vi "Debugger_Application.vi"() -> ()   [LabVIEW 2016]
uses:
  Z:/original_project/CodeConverter/Controls/CommandLine.ctl
  Z:/original_project/CodeConverter/Controls/EX.Command.ctl
  Z:/original_project/CodeConverter/Controls/WB.Operation.ctl
  Z:/original_project/CodeConverter/SoftCoreCodeConverter.lvlib
panel:
  out "Instruction stop":bool
  in  "Breakpoint signal":bool
  in  "Breakpoint control":i32
  in  "Run":bool
  out "Instruction Number":i32=7
  in  "Breakpoint On/Off":bool
  in  "Instruction Step Mode":bool
  in  "Instruction  Delay":u32=100
  out "Current Output /Ins":dbl
  out "DataMemory Out":dbl[](array[numeric])=[0.0, 1.0, 2.0, 3.0, 4.0, 5.0, 6.0, 7.0, 8.0, 9.0, 10.0, 11.0, 15.0, 16.0, 17.0, 18.0, 19.0, 20.0, 0.0, 0.0, 0.0, 0.0, 0.0, 0.0, 0.0, 0.0, 0.0, 0.0, 0.0, 0.0, 0.0, 0.0, 0.0, 0.0, 0.0, 0.0, 0.0, 0.0, 0.0, 0.0, 0.0, 0.0, 0.0, 0.0, 0.0, 0.0, 0.0, 0.0, 0.0, 0.0, 0.0, 0.0, 0.0, 0.0, 0.0, 0.0, 0.0, 0.0, 0.0, 0.0, 0.0, 0.0, 0.0, 0.0, 0.0, 0.0, 0.0, 0.0, 0.0, 0.0, 0.0, 0.0, 0.0, 0.0, 0.0, 0.0, 0.0, 0.0, 0.0, 0.0, 0.0, 0.0, 0.0, 0.0, 0.0, 0.0, 0.0, 0.0, 0.0, 0.0, 0.0, 0.0, 0.0, 0.0, 0.0, 0.0, 0.0, 0.0, 0.0, 0.0, 0.0, 0.0, 0.0, 0.0, 0.0, 0.0, 0.0, 0.0, 0.0, 0.0, 0.0, 0.0, 0.0, 0.0, 0.0, 0.0, 0.0, 0.0, 0.0, 0.0, 0.0, 0.0, 0.0, 0.0, 0.0, 0.0, 0.0, 0.0, 0.0, 0.0, 0.0, 0.0, 0.0, 0.0, 0.0, 0.0, 0.0, 0.0, 0.0, 0.0, 0.0, 0.0, 0.0, 0.0, 0.0, 0.0, 0.0, 0.0, 0.0, 0.0, 0.0, 0.0, 0.0, 0.0, 0.0, 0.0, 0.0, 0.0, 0.0, 0.0, 0.0, 0.0, 0.0, 0.0, 0.0, 0.0, 0.0, 0.0, 0.0, 0.0, 0.0, 0.0, 0.0, 0.0, 0.0, 0.0, 0.0, 0.0, 0.0, 0.0, 0.0, 0.0, 0.0, 0.0, 0.0, 0.0, 0.0, 0.0, 0.0, 0.0, 0.0, 0.0, 0.0, 0.0, 0.0, 0.0, 0.0, 0.0, 0.0, 0.0, 0.0, 0.0, 0.0, 0.0, 0.0, 0.0, 0.0, 0.0, 0.0, 0.0, 0.0, 0.0, 0.0, 0.0, 0.0, 0.0, 0.0, 0.0, 0.0, 0.0, 0.0, 0.0, 0.0, 0.0, 0.0, 0.0, 0.0, 0.0, 0.0, 0.0, 0.0, 0.0, 0.0, 0.0, 0.0, 0.0, 0.0, 0.0, 0.0, 0.0, 0.0, 0.0, 0.0, 0.0, 0.0, 0.0, 0.0, 0.0, 0.0, 0.0, 0.0, 0.0, 0.0, 0.0, 0.0]
  out "Current Operation":T1=enum."None"
  out "Output array":dbl[](array[numeric])
  in  "Input":dbl[](array[numeric])=[0.0, 15.0, 20.0, 3.0, 4.0, 5.0, 6.0, 7.0, 8.0, 9.0, 10.0, 11.0, 15.0, 16.0, 17.0, 18.0, 19.0, 20.0, 0.0, 0.0, 0.0, 0.0, 0.0, 0.0, 0.0, 0.0, 0.0, 0.0, 0.0, 0.0, 0.0, 0.0, 0.0, 0.0, 0.0, 0.0, 0.0, 0.0, 0.0, 0.0, 0.0, 0.0, 0.0, 0.0, 0.0, 0.0, 0.0, 0.0, 0.0, 0.0, 0.0, 0.0, 0.0, 0.0, 0.0, 0.0, 0.0, 0.0, 0.0, 0.0, 0.0, 0.0, 0.0, 0.0, 0.0, 0.0, 0.0, 0.0, 0.0, 0.0, 0.0, 0.0, 0.0, 0.0, 0.0, 0.0, 0.0, 0.0, 0.0, 0.0, 0.0, 0.0, 0.0, 0.0, 0.0, 0.0, 0.0, 0.0, 0.0, 0.0, 0.0, 0.0, 0.0, 0.0, 0.0, 0.0, 0.0, 0.0, 0.0, 0.0, 0.0, 0.0, 0.0, 0.0, 0.0, 0.0, 0.0, 0.0, 0.0, 0.0, 0.0, 0.0, 0.0, 0.0, 0.0, 0.0, 0.0, 0.0, 0.0, 0.0, 0.0, 0.0, 0.0, 0.0, 0.0, 0.0, 0.0, 0.0, 0.0, 0.0, 0.0, 0.0, 0.0, 0.0, 0.0, 0.0, 0.0, 0.0, 0.0, 0.0, 0.0, 0.0, 0.0, 0.0, 0.0, 0.0, 0.0, 0.0, 0.0, 0.0, 0.0, 0.0, 0.0, 0.0, 0.0, 0.0, 0.0, 0.0, 0.0, 0.0, 0.0, 0.0, 0.0, 0.0, 0.0, 0.0, 0.0, 0.0, 0.0, 0.0, 0.0, 0.0, 0.0, 0.0, 0.0, 0.0, 0.0, 0.0, 0.0, 0.0, 0.0, 0.0, 0.0, 0.0, 0.0, 0.0, 0.0, 0.0, 0.0, 0.0, 0.0, 0.0, 0.0, 0.0, 0.0, 0.0, 0.0, 0.0, 0.0, 0.0, 0.0, 0.0, 0.0, 0.0, 0.0, 0.0, 0.0, 0.0, 0.0, 0.0, 0.0, 0.0, 0.0, 0.0, 0.0, 0.0, 0.0, 0.0, 0.0, 0.0, 0.0, 0.0, 0.0, 0.0, 0.0, 0.0, 0.0, 0.0, 0.0, 0.0, 0.0, 0.0, 0.0, 0.0, 0.0, 0.0, 0.0, 0.0, 0.0, 0.0, 0.0, 0.0, 0.0, 0.0, 0.0, 0.0, 0.0, 0.0, 0.0, 0.0, 0.0, 0.0, 0.0, 0.0, 0.0]
  out "Loop Mode Iteration":i32
  in  "Loop Delay":u32=1000
  in  "Loop Step Mode":bool
  in  "Loop Mode":bool
  in  "DataMemory Input":dbl[](array[numeric])=[0.0, 1.0, 2.0, 3.0, 4.0, 5.0, 6.0, 7.0, 8.0, 9.0, 10.0, 11.0, 15.0, 16.0, 17.0, 18.0, 19.0, 20.0, 0.0, 0.0, 0.0, 0.0, 0.0, 0.0, 0.0, 0.0, 0.0, 0.0, 0.0, 0.0, 0.0, 0.0, 0.0, 0.0, 0.0, 0.0, 0.0, 0.0, 0.0, 0.0, 0.0, 0.0, 0.0, 0.0, 0.0, 0.0, 0.0, 0.0, 0.0, 0.0, 0.0, 0.0, 0.0, 0.0, 0.0, 0.0, 0.0, 0.0, 0.0, 0.0, 0.0, 0.0, 0.0, 0.0, 0.0, 0.0, 0.0, 0.0, 0.0, 0.0, 0.0, 0.0, 0.0, 0.0, 0.0, 0.0, 0.0, 0.0, 0.0, 0.0, 0.0, 0.0, 0.0, 0.0, 0.0, 0.0, 0.0, 0.0, 0.0, 0.0, 0.0, 0.0, 0.0, 0.0, 0.0, 0.0, 0.0, 0.0, 0.0, 0.0, 0.0, 0.0, 0.0, 0.0, 0.0, 0.0, 0.0, 0.0, 0.0, 0.0, 0.0, 0.0, 0.0, 0.0, 0.0, 0.0, 0.0, 0.0, 0.0, 0.0, 0.0, 0.0, 0.0, 0.0, 0.0, 0.0, 0.0, 0.0, 0.0, 0.0, 0.0, 0.0, 0.0, 0.0, 0.0, 0.0, 0.0, 0.0, 0.0, 0.0, 0.0, 0.0, 0.0, 0.0, 0.0, 0.0, 0.0, 0.0, 0.0, 0.0, 0.0, 0.0, 0.0, 0.0, 0.0, 0.0, 0.0, 0.0, 0.0, 0.0, 0.0, 0.0, 0.0, 0.0, 0.0, 0.0, 0.0, 0.0, 0.0, 0.0, 0.0, 0.0, 0.0, 0.0, 0.0, 0.0, 0.0, 0.0, 0.0, 0.0, 0.0, 0.0, 0.0, 0.0, 0.0, 0.0, 0.0, 0.0, 0.0, 0.0, 0.0, 0.0, 0.0, 0.0, 0.0, 0.0, 0.0, 0.0, 0.0, 0.0, 0.0, 0.0, 0.0, 0.0, 0.0, 0.0, 0.0, 0.0, 0.0, 0.0, 0.0, 0.0, 0.0, 0.0, 0.0, 0.0, 0.0, 0.0, 0.0, 0.0, 0.0, 0.0, 0.0, 0.0, 0.0, 0.0, 0.0, 0.0, 0.0, 0.0, 0.0, 0.0, 0.0, 0.0, 0.0, 0.0, 0.0, 0.0, 0.0, 0.0, 0.0, 0.0, 0.0, 0.0, 0.0, 0.0, 0.0, 0.0, 0.0, 0.0, 0.0, 0.0, 0.0, 0.0, 0.0]
  in  "CoreCode":T2[][](array[typedef])=[[{"Ex.Command"=enum."None", "Ex.AddressIn1"=1.0, "Ex.AddressIn2"=0.0, "WB.Command"=enum."In", "WB.AddressOut"=3.0, "Bypass1"=0.0, "Bypass 2"=0.0}], [{"Ex.Command"=enum."None", "Ex.AddressIn1"=2.0, "Ex.AddressIn2"=0.0, "WB.Command"=enum."In", "WB.AddressOut"=4.0, "Bypass1"=0.0, "Bypass 2"=0.0}], [{"Ex.Command"=enum."None", "Ex.AddressIn1"=3.0, "Ex.AddressIn2"=4.0, "WB.Command"=enum."Mul", "WB.AddressOut"=5.0, "Bypass1"=0.0, "Bypass 2"=0.0}], [{"Ex.Command"=enum."None", "Ex.AddressIn1"=5.0, "Ex.AddressIn2"=0.0, "WB.Command"=enum."Mov", "WB.AddressOut"=6.0, "Bypass1"=0.0, "Bypass 2"=0.0}], [{"Ex.Command"=enum."None", "Ex.AddressIn1"=6.0, "Ex.AddressIn2"=0.0, "WB.Command"=enum."Out", "WB.AddressOut"=3.0, "Bypass1"=0.0, "Bypass 2"=0.0}], [{"Ex.Command"=enum."None", "Ex.AddressIn1"=0.0, "Ex.AddressIn2"=0.0, "WB.Command"=enum."None", "WB.AddressOut"=0.0, "Bypass1"=0.0, "Bypass 2"=0.0}], [{"Ex.Command"=enum."None", "Ex.AddressIn1"=0.0, "Ex.AddressIn2"=0.0, "WB.Command"=enum."None", "WB.AddressOut"=0.0, "Bypass1"=0.0, "Bypass 2"=0.0}], [{"Ex.Command"=enum."None", "Ex.AddressIn1"=5.0, "Ex.AddressIn2"=9.0, "WB.Command"=enum."None", "WB.AddressOut"=0.0, "Bypass1"=0.0, "Bypass 2"=0.0}]]
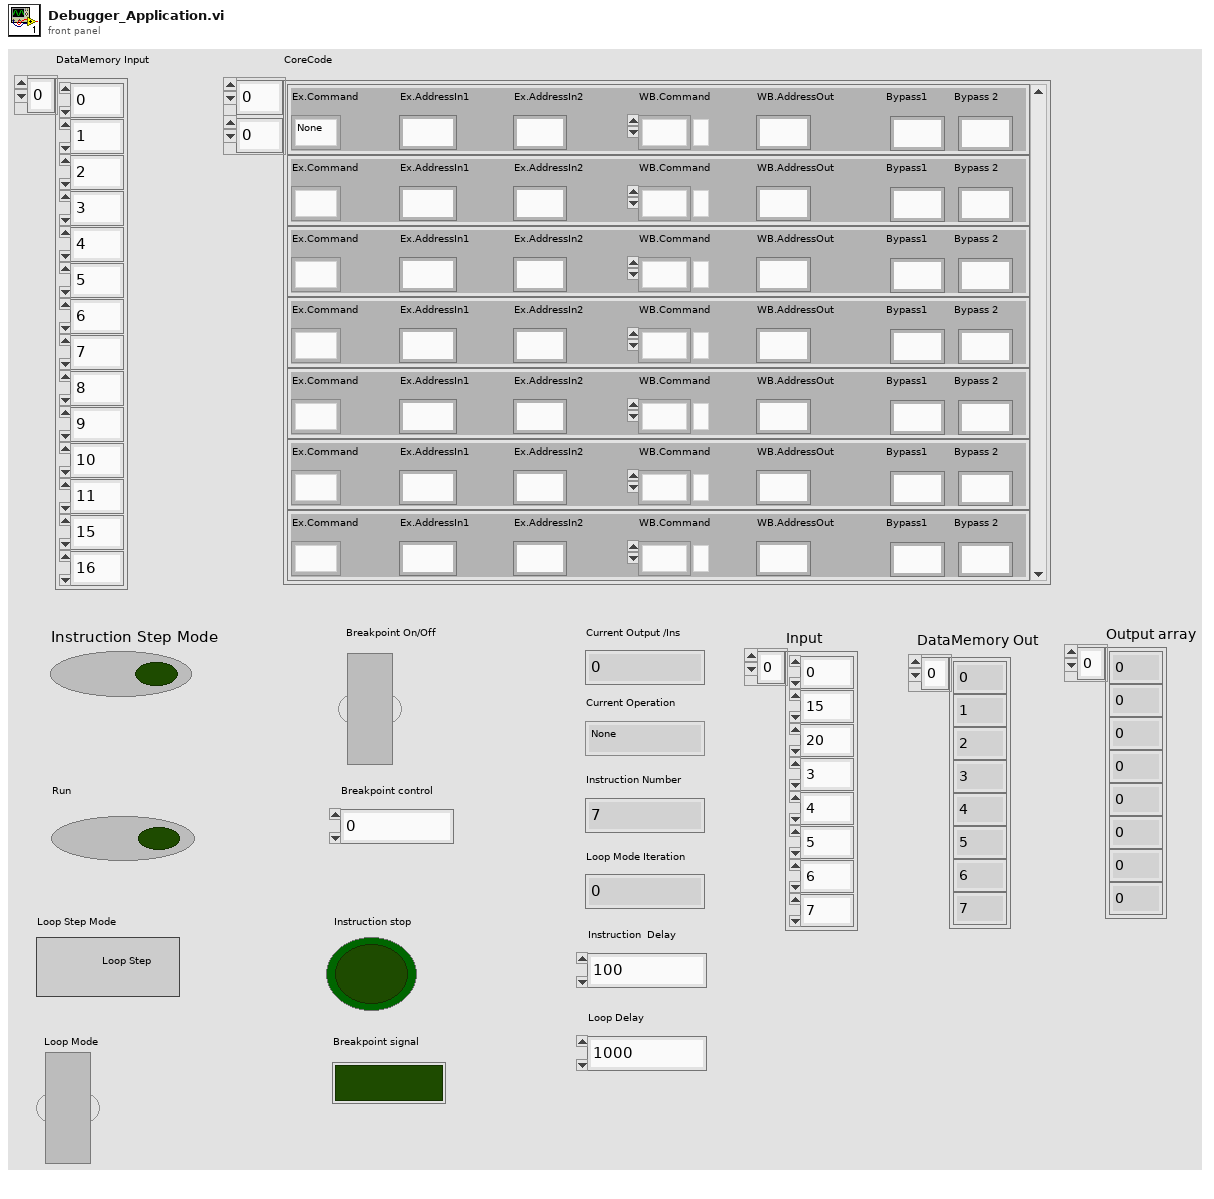
[diagram p1: front panel]
types:
  T1 = typedef "SoftCoreCodeConverter.lvlib/WB.Operation.ctl" = enum8{"In", "Out", "Mov", "Add", "Sub", "Mul", "Div", "None", "Sqr", "Sin", "Cos", "Sgl2Dbl", "Dbl2Int", "Int2Dbl", "Mlookup", "Dbl2Sgl", "G_IsPOS", "G_IsNEG", "G_IsNULL", "G_IsNNULL", "G_IsNAN", "G_IsNNAN", "G_IsIFTY", "G_IsNIFTY", "reserved_0", "reserved_1", "reserved_2", "reserved_3", "reserved_4", "reserved_5", "reserved_6", "reserved_7"}
  T2 = typedef "SoftCoreCodeConverter.lvlib/CommandLine.ctl" = cluster{"Ex.Command":T3, "Ex.AddressIn1":fxp<+,16,16>, "Ex.AddressIn2":fxp<+,16,16>, "WB.Command":T1, "WB.AddressOut":fxp<+,16,16>, "Bypass1":fxp<+,2,2>, "Bypass 2":fxp<+,2,2>}
  T3 = typedef "SoftCoreCodeConverter.lvlib/EX.Command.ctl" = enum8{"Default", "Sub", "None", "Fuse", "Abs", "AbsSub", "Const"}
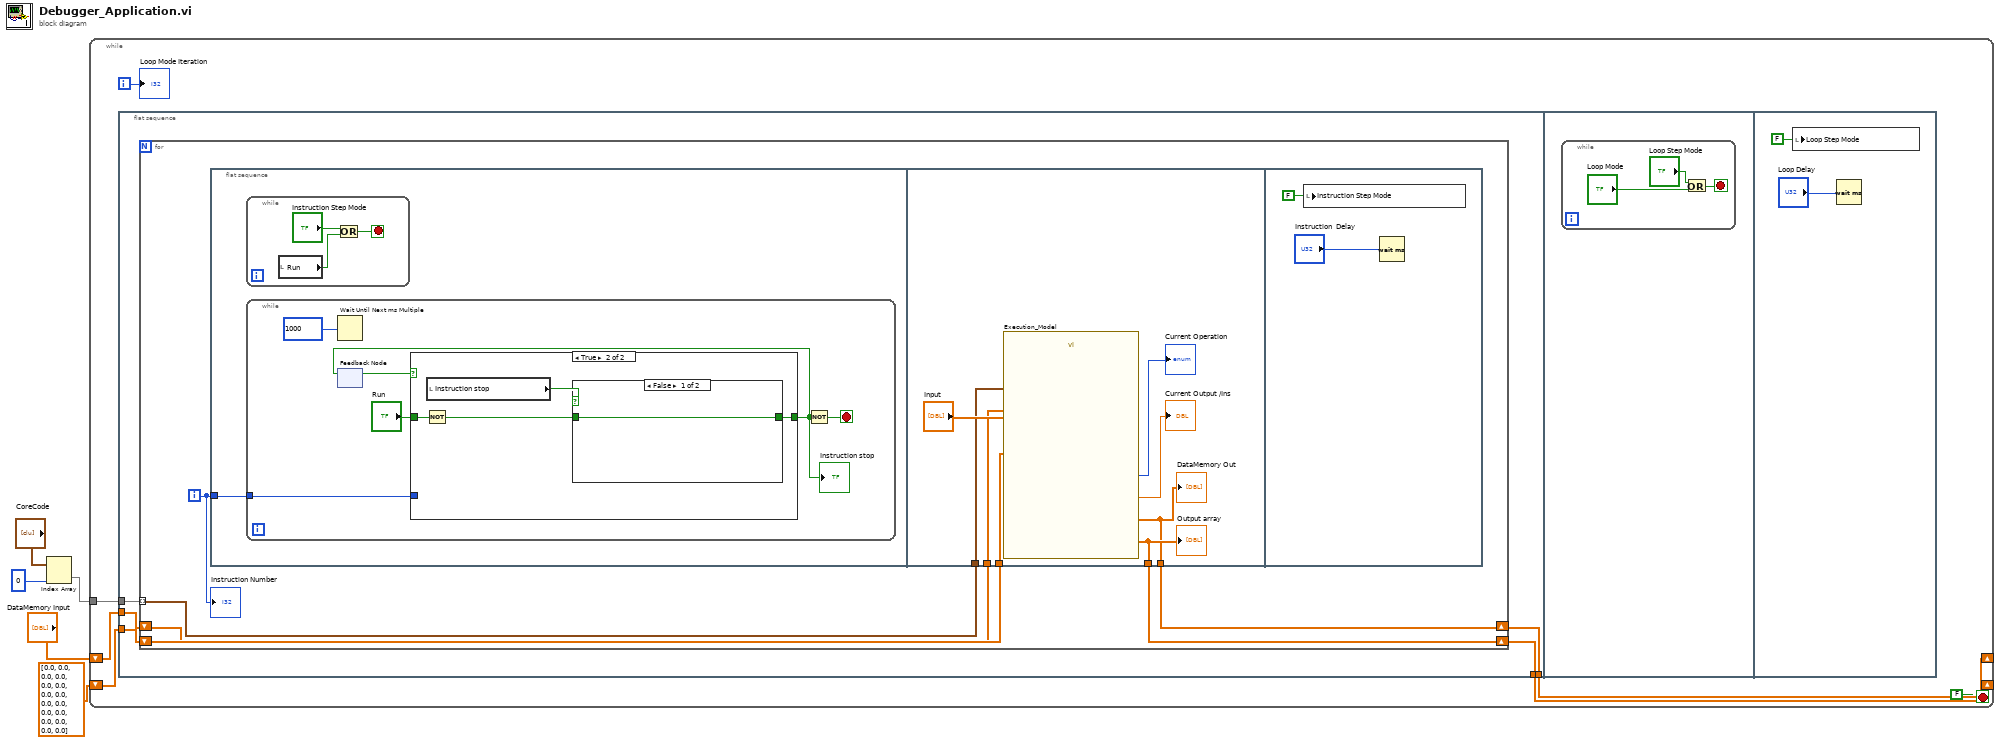
[diagram p0: block diagram]
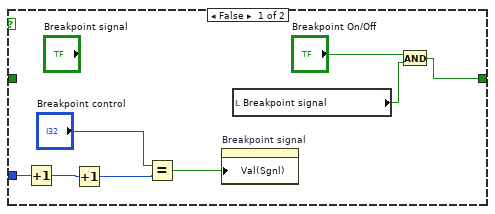
[diagram p2: hidden frame]
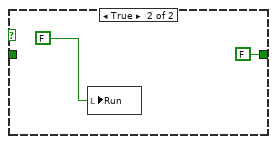
[diagram p3: hidden frame]
diagram:
  n1 = Index Array(array="CoreCode", index (col)=0 ("disabled index (col)")) -> (element=w3:T2[])  [unwired: 1 in]
  n2 = while {
    tunnel: w3 -> [w12]
    shift-right: [w8] -> _
    shift-left: "DataMemory Input" -> [w11]
    shift-right: [w9] -> _
    shift-left: dbl[] [0.0, 0.0, 0.0, 0.0, 0.0, 0.0, 0.0, 0.0, 0.0, 0.0, 0.0, 0.0, 0.0, 0.0, 0.0, 0.0] ("output array") -> [w10]
    i -> [w6]
    stop <- FALSE stop-if-true
    n3 = flat-sequence {
      tunnel: w12 -> [w17]
      tunnel: w11 -> [w16]
      tunnel: w10 -> [w15]
      tunnel: [w14] -> w9
      tunnel: [w13] -> w8
      frame #0 {
        n4 = for {
          shift-right: [w19] -> w13
          shift-left: w16 -> [w21]
          shift-right: [w20] -> w14
          shift-left: w15 -> [w23]
          tunnel: w17 -> [w22] mode=indexing
          i -> [w18]
          n5 = flat-sequence {
            tunnel: w18 -> [w24]
            tunnel: w23 -> [w55]
            tunnel: w22 -> [w54]
            tunnel: w21 -> [w53]
            tunnel: [w50] -> w20
            tunnel: [w49] -> w19
            frame #0 {
              n6 = while {
                stop <- w25 stop-if-true
                n7 = local read "Run"() -> (w27:bool)
                n8 = Or(x="Instruction Step Mode", y=w27) -> (x .or. y?=w25:bool)
              }
              n9 = while {
                tunnel: w24 -> [w33]
                stop <- w31 stop-if-true
                n10 = Wait Until Next ms Multiple(millisecond multiple=u32 1000) -> ()  [unwired: 1 out]
                n11 = feedback #1() -> (w32:bool)  [unwired: 1 in]
                n12 = case shown="True" w32 {
                  tunnel: w33 -> [w38 _]
                  tunnel: [w36 w45] -> w28
                  tunnel: "Run" -> [_ w44]
                  frame False {
                    n13 = Increment(x=w38) -> (x+1=w35:i32)
                    n14 = Increment(x=w35) -> (x+1=w34:i32)
                    n15 = Equal?(x="Breakpoint control", y=w34) -> (x = y?=w40:bool)
                    n16 = property on="Breakpoint signal" class="Bool (strict)"("Val(Sgnl)"=w40) -> ()  [unwired: 2 in, 2 out]
                    n17 = local read "Breakpoint signal"() -> (w39:bool)
                    n18 = And(x="Breakpoint On/Off", y=w39) -> (x .and. y?=w36:bool)
                  }
                  frame True {
                    n19 = Not(x=w44) -> (.not. x?=w43:bool)
                    n20 = local read "Instruction stop"() -> (w42:bool)
                    n21 = case shown="False" w42 {
                      tunnel: [w46 FALSE] -> w45
                      tunnel: w43 -> [w46 _]
                      frame False {
                      }
                      frame True {
                        n22 = local write "Run"(FALSE) -> ()
                      }
                    }
                  }
                }
                "Instruction stop" <- w28
                n23 = feedback-in #1(w28) -> ()
                n24 = Not(x=w28) -> (.not. x?=w31:bool)
              }
            }
            frame #1 {
              n25 = call "Execution_Model.vi"("output array 3"=w55, "Input"="Input", "CodeLine"=w54, "DataMemory Input"=w53) -> ("output array"=w50:dbl[], "DataMemory Out"=w49:dbl[], "Current Output /Ins"=→"Current Output /Ins":dbl, "Curren Operation"=→"Current Operation":T1)  [unwired: 2 in, 2 out]
              "DataMemory Out" <- w49
              "Output array" <- w50
            }
            frame #2 {
              n26 = local write "Instruction Step Mode"(FALSE ("Step")) -> ()
              n27 = Wait (ms)(milliseconds to wait="Instruction  Delay") -> ()  [unwired: 1 out]
            }
          }
          "Instruction Number" <- w18
        }
      }
      frame #1 {
        n28 = while {
          stop <- w60 stop-if-true
          n29 = Or(x="Loop Step Mode", y="Loop Mode") -> (x .or. y?=w60:bool)
        }
      }
      frame #2 {
        n30 = local write "Loop Step Mode"(FALSE ("Step 2")) -> ()
        n31 = Wait (ms)(milliseconds to wait="Loop Delay") -> ()  [unwired: 1 out]
      }
    }
    "Loop Mode Iteration" <- w6
  }
